vi "抽奖.vi"() -> ()   [LabVIEW 2025]
panel:
  in  "清空":bool
  in  "清空":dbl[](array[numeric])
  out "被抽中的人的序号":dbl[](array[numeric])=[21.0, 2.0, 15.0, 5.0, 20.0, 22.0, 19.0, 13.0, 16.0]
  in  "参与者":string[](array[string])=["李白", "杜甫", "ËÕéø", "苏辙", "ËÕä­", "白居易", "王维", "李清照", "韩愈", "柳宗元", "陶渊明", "曾巩", "黄耀荣", "骆宾王", "欧阳修", "高适", "李贺", "屈原", "辛弃疾", "陆游", "贺知章", "刘禹锡"]
  out "一等奖":string[](array[string])=["黄耀荣", "高适"]
  out "二等奖":string[](array[string])=["陆游", "刘禹锡", "辛弃疾"]
  out "三等奖":string[](array[string])=["贺知章", "杜甫", "欧阳修", "ËÕä­"]
  in  "参与抽奖人数":dbl=22.0
  in  "开始抽奖":bool
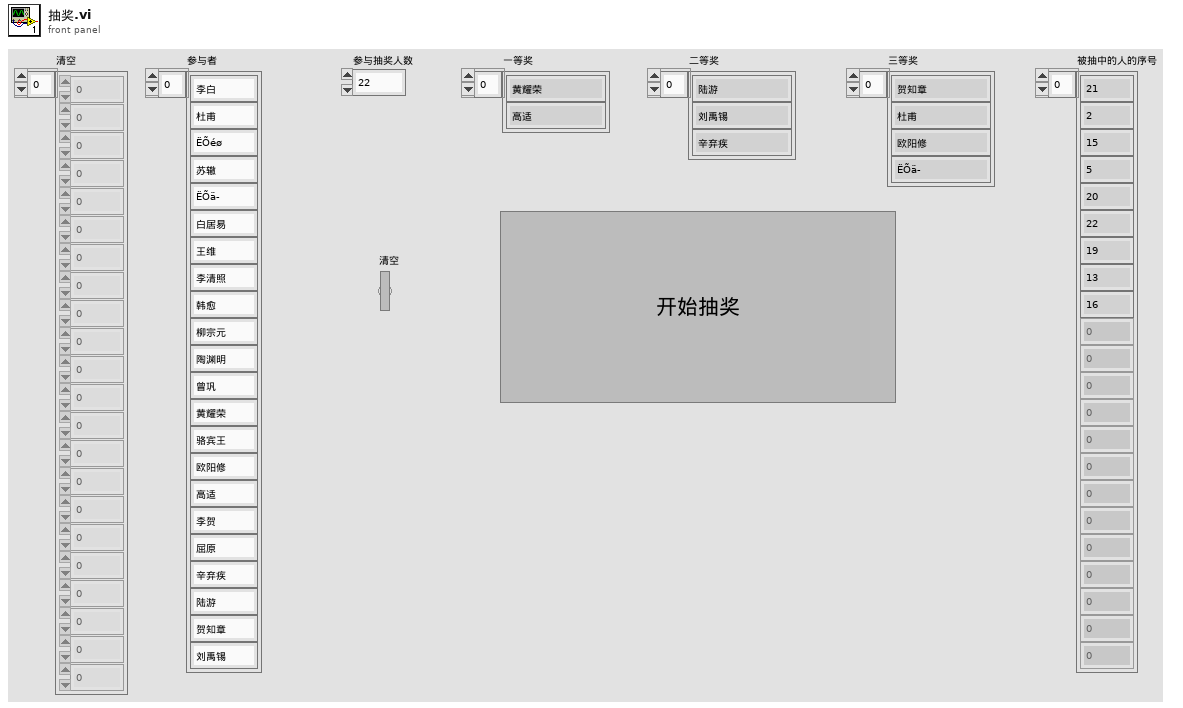
[diagram p1: front panel]
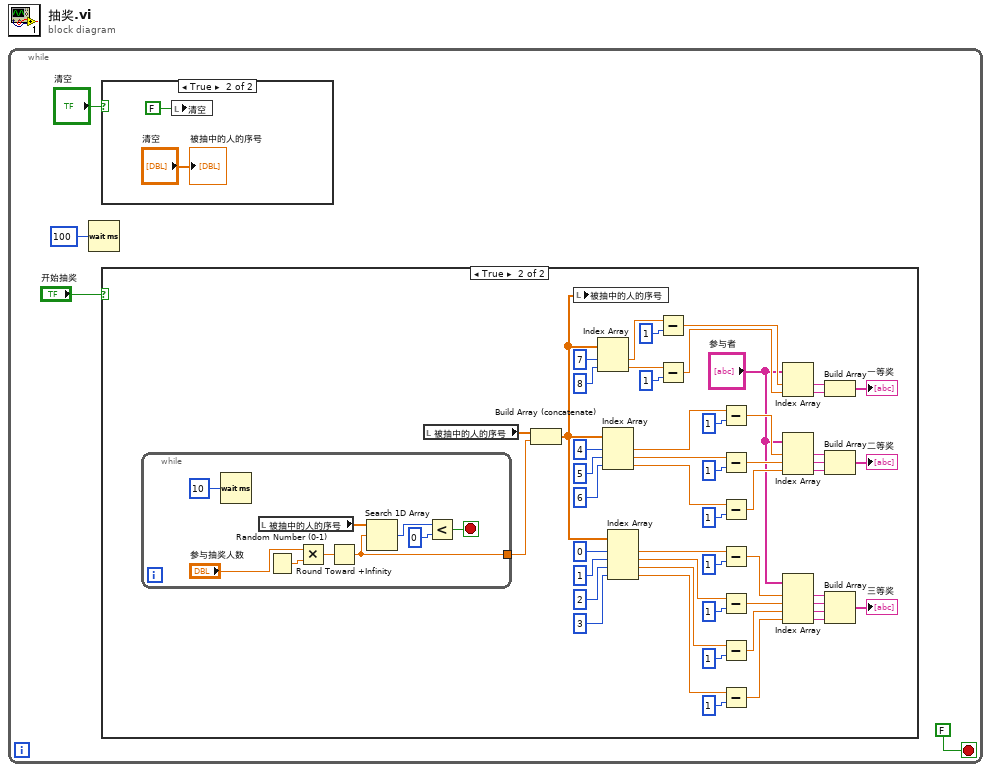
[diagram p0: block diagram]
diagram:
  n1 = while {
    stop <- FALSE stop-if-true
    n2 = Wait (ms)(milliseconds to wait=u32 100 ("毫秒计时值")) -> ()  [unwired: 1 out]
    n3 = case shown="True" "清空" {
      frame False {
      }
      frame True {
        n4 = local write "清空"(FALSE ("清空 2")) -> ()
        "被抽中的人的序号" <- "清空"
      }
    }
    n5 = case shown="True" "开始抽奖" {
      frame False {
      }
      frame True {
        n6 = while {
          tunnel: [w60] -> w9
          stop <- w65 stop-if-true
          n7 = Wait (ms)(milliseconds to wait=u32 10 ("毫秒计时值")) -> ()  [unwired: 1 out]
          n8 = local read "被抽中的人的序号"() -> (w59:dbl[])
          n9 = Random Number (0-1)() -> (number: 0 to 1=w63:dbl)
          n10 = Multiply(x="参与抽奖人数", y=w63) -> (x*y=w64:dbl)
          n11 = Round Toward +Infinity(x=w64) -> (ceil(x): smallest int >= x=w60:dbl)
          n12 = Search 1D Array(1D array=w59, element=w60) -> (index of element=w67:i32)  [unwired: 1 in]
          n13 = Less?(x=w67, y=0) -> (x < y?=w65:bool)
        }
        n14 = local read "被抽中的人的序号"() -> (w8:dbl[])
        n15 = Build Array (concatenate)(w8, w9) -> (w7:dbl[])
        n16 = local write "被抽中的人的序号"(w7) -> ()
        n17 = Index Array(array=w7, index #1=7, index #2=8) -> (element #1=w48:dbl, element #2=w46:dbl)
        n18 = Index Array(array=w7, index #1=4, index #2=5, index #3=6) -> (element #1=w44:dbl, element #2=w42:dbl, element #3=w40:dbl)
        n19 = Index Array(array=w7, index #1=0, index #2=1, index #3=2, index #4=3) -> (element #1=w35:dbl, element #2=w34:dbl, element #3=w33:dbl, element #4=w32:dbl)
        n20 = Subtract(x=w48, y=1) -> (x-y=w58:dbl)
        n21 = Subtract(x=w46, y=1) -> (x-y=w57:dbl)
        n22 = Subtract(x=w44, y=1) -> (x-y=w56:dbl)
        n23 = Subtract(x=w42, y=1) -> (x-y=w55:dbl)
        n24 = Subtract(x=w40, y=1) -> (x-y=w54:dbl)
        n25 = Subtract(x=w35, y=1) -> (x-y=w53:dbl)
        n26 = Subtract(x=w34, y=1) -> (x-y=w52:dbl)
        n27 = Subtract(x=w33, y=1) -> (x-y=w51:dbl)
        n28 = Subtract(x=w32, y=1) -> (x-y=w50:dbl)
        n29 = Index Array(array="参与者", index #1=w58, index #2=w57) -> (element #1=w30:string, element #2=w29:string)
        n30 = Index Array(array="参与者", index #1=w56, index #2=w55, index #3=w54) -> (element #1=w22:string, element #2=w23:string, element #3=w24:string)
        n31 = Index Array(array="参与者", index #1=w53, index #2=w52, index #3=w51, index #4=w50) -> (element #1=w28:string, element #2=w27:string, element #3=w26:string, element #4=w25:string)
        n32 = Build Array(w30, w29) -> (→"一等奖":string[])
        n33 = Build Array(w22, w23, w24) -> (→"二等奖":string[])
        n34 = Build Array(w28, w27, w26, w25) -> (→"三等奖":string[])
      }
    }
  }
